vi "Draw Arrow at Bearing for arrow.vi"(4 "pen":T1={"Width"=1, "Style"=enum."Solid"}, 6 "color(black)":u32(colorbox), 9 "P2":cluster{"Horizontal":i32, "Vertical":i32}, 10 "P1":cluster{"Horizontal":i32, "Vertical":i32}, 11 "new picture in":picture) -> (3 "new picture out":picture)   [LabVIEW 2020, in "GarphView.lvlib" / "GarphView.lvclass"]
uses:
  GarphView.lvclass
panel:
  out "Degrees":dbl
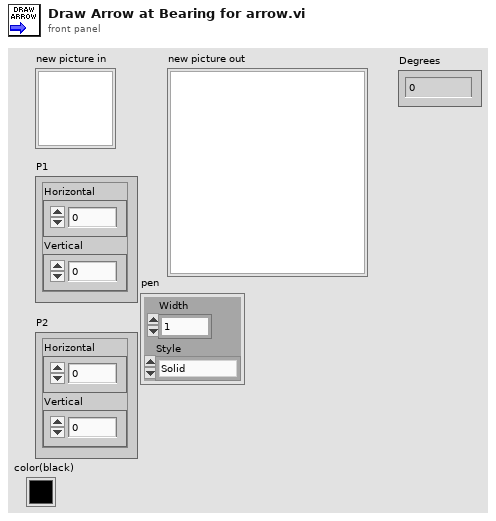
[diagram p1: front panel]
types:
  T1 = cluster{"Width":u16, "Style":enum32{"Solid", "Dash", "Dot", "DashDot", "DashDotDot"}}
  T2 = enum32{"Solid", "Dash", "Dot", "DashDot", "DashDotDot"}
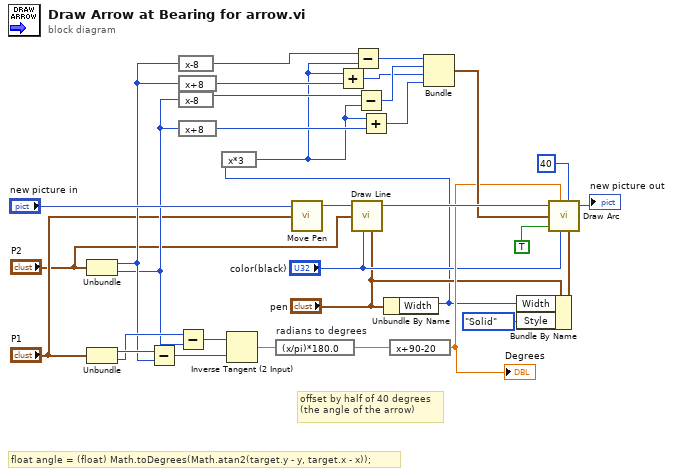
[diagram p0: block diagram]
diagram:
  # "offset by half of 40 degrees\n(the angle of the arrow)"
  # "float angle = (float) Math.toDegrees(Math.atan2(target.y - y, target.x - x));"
  n1 = Unbundle("P2") -> ("Horizontal"=w22:i32, "Vertical"=w21:i32)
  n2 = Unbundle("P1") -> ("Horizontal"=w32:i32, "Vertical"=w30:i32)
  n3 = Subtract(x=w32, y=w22) -> (x-y=w31:i32)
  n4 = Subtract(x=w30, y=w21) -> (x-y=w29:i32)
  n5 = expression code="x-8"(w22) -> (w20:i32)
  n6 = expression code="x+8"(w22) -> (w18:i32)
  n7 = expression code="x-8"(w21) -> (w17:i32)
  n8 = expression code="x+8"(w21) -> (w16:i32)
  n9 = Inverse Tangent (2 Input)(1:w31, 2:w29) -> (0:w28:dbl)
  n10 = expression code="(x/pi)*180.0" "radians to degrees"(w28) -> (w15:dbl)
  n11 = call <vilib>:"Move Pen.vi"("new position"="P1", "picture"="new picture in") -> ("new picture"=w13:picture)  [unwired: 3 in]
  n12 = call <vilib>:"Draw Line.vi"("picture"=w13, "end point"="P2", "color(black)"="color(black)", "pen"="pen") -> ("new picture"=w25:picture)  [unwired: 5 in]
  n13 = Unbundle By Name("pen") -> ("Width"=w1:u16)
  n14 = expression code="x*3" ("radians to degrees")(w1) -> (w2:u16)
  n15 = Add(x=w2, y=w18) -> (x+y=w3:i32)
  n16 = Subtract(x=w20, y=w2) -> (x-y=w6:i32)
  n17 = Subtract(x=w17, y=w2) -> (x-y=w5:i32)
  n18 = Add(x=w2, y=w16) -> (x+y=w4:i32)
  n19 = expression code="x+90-20" ("radians to degrees")(w15) -> (w14:dbl)
  "Degrees" <- w14
  n20 = Bundle(w6, w5, w3, w4) -> (w19:cluster{i32, i32, i32, i32})  [unwired: 1 in]
  n21 = Bundle By Name(cluster="pen", "Width"=w1, "Style"=T2."Solid") -> (w7:T1)
  n22 = call <vilib>:"Draw Arc.vi"("picture"=w25, "start angle[degrees]"=w14, "rect"=w19, "fill?(F)"=TRUE, "color(black)"="color(black)", "arc size[degrees]"=i16 40, "pen"=w7) -> ("new picture"=→"new picture out":picture)  [unwired: 2 in]
